vi "Disable GUI Objects inside SomeTemplatesFound Tab.vi"(8 "error in":errorcluster, 11 "GUI Objects":T1) -> (0 "error out":errorcluster)   [LabVIEW 2022 SP3]
doc: "Disables and greyes out all the GUI objects found inside the \"SomeTemplatesFound\" page of the Tab Control."
uses:
  GUI Object Refs (cluster).ctl
panel:
  # "Development\ncontrols/indicators useful for development and testing, but which are not outputs of the VI"
  # "Input\nInputs to the VI"
  # "Output\nOutputs of the VI"
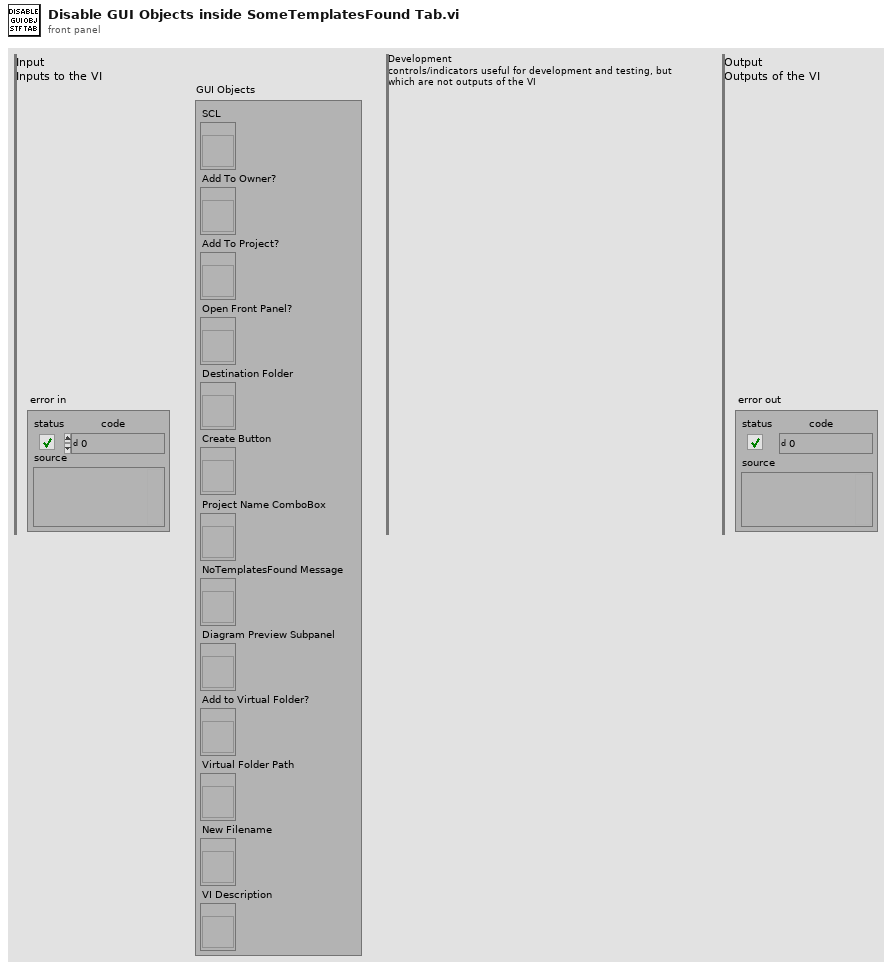
[diagram p1: front panel]
types:
  T1 = typedef "GUI Object Refs (cluster).ctl" = cluster{"SCL":refnum<vi>, "Add To Owner?":refnum<vi>, "Add To Project?":refnum<vi>, "Open Front Panel?":refnum<vi>, "Destination Folder":refnum<vi>, "Create Button":refnum<vi>, "Project Name ComboBox":refnum<vi>, "NoTemplatesFound Message":refnum<vi>, "Diagram Preview Subpanel":refnum<vi>, "Add to Virtual Folder?":refnum<vi>, "Virtual Folder Path":refnum<vi>, "New Filename":refnum<vi>, "VI Description":refnum<vi>}
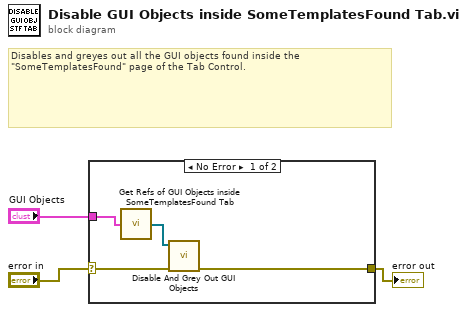
[diagram p0: block diagram]
diagram:
  # "Disables and greyes out all the GUI objects found inside the \"SomeTemplatesFound\" page of the Tab Control."
  n1 = case shown="No Error" "error in" {
    selector: "error in" -> [w5 w8]
    tunnel: [w6 w8] -> w2
    tunnel: "GUI Objects" -> [w7 _]
    frame No Error {
      n2 = call "Get Refs of GUI Objects inside SomeTemplatesFound Tab.vi"("GUI Objects"=w7) -> ("Refs of GUI Objects inside SomeTemplatesFound Tab"=w4:refnum<vi>[])
      n3 = call "Disable And Grey Out GUI Objects.vi"("Error In"=w5, "GUI Object Refs"=w4) -> ("Error Out"=w6:errorcluster)  [unwired: 9 in]
    }
    frame Error {
    }
  }
  "error out" <- w2
